vi "HW_7p1_Task2_nguyejk.vi"() -> ()   [LabVIEW 2016]
panel:
  out "Hypotension":dbl
  out "Normal":dbl
  out "Hypertension":dbl
  in  "Numeric":i32
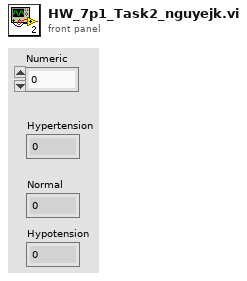
[diagram p1: front panel]
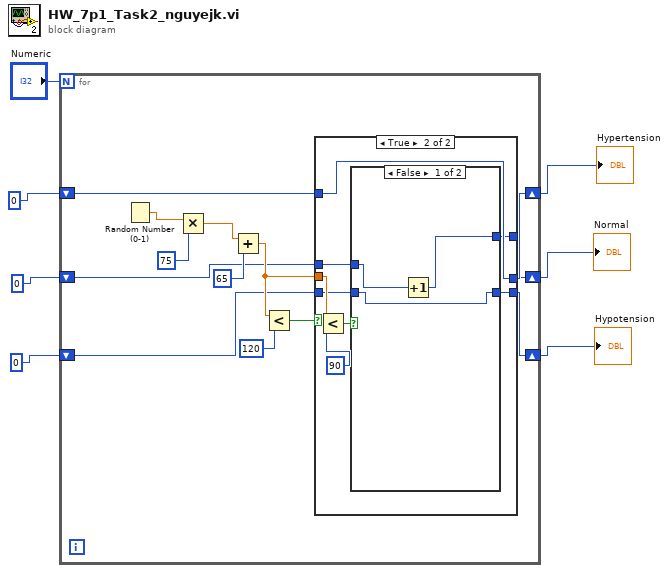
[diagram p0: block diagram]
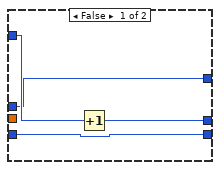
[diagram p2: hidden frame]
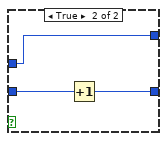
[diagram p3: hidden frame]
diagram:
  n1 = for {
    N: "Numeric" -> [_]
    shift-right: [w14] -> w4
    shift-left: 0 -> [w12]
    shift-right: [w11] -> w5
    shift-left: 0 -> [w10]
    shift-right: [w9] -> w1
    shift-left: 0 -> [w8]
    n2 = Random Number (0-1)() -> (number: 0 to 1=w17:dbl)
    n3 = Multiply(x=w17, y=75) -> (x*y=w19:dbl)
    n4 = Add(x=w19, y=65) -> (x+y=w13:dbl)
    n5 = Less?(x=w13, y=120) -> (x < y?=w16:bool)
    n6 = case shown="True" w16 {
      tunnel: [w24 w29] -> w14
      tunnel: w13 -> [_ w31]
      tunnel: w12 -> [w23 w29]
      tunnel: [w21 w28] -> w11
      tunnel: w10 -> [w21 w27]
      tunnel: [w22 w26] -> w9
      tunnel: w8 -> [w22 w25]
      frame False {
        n7 = Increment(x=w23) -> (x+1=w24:i32)
      }
      frame True {
        n8 = Less?(x=w31, y=90) -> (x < y?=w30:bool)
        n9 = case shown="False" w30 {
          tunnel: [w33 w38] -> w28
          tunnel: w27 -> [w33 w37]
          tunnel: [w35 w36] -> w26
          tunnel: w25 -> [w34 w36]
          frame False {
            n10 = Increment(x=w34) -> (x+1=w35:i32)
          }
          frame True {
            n11 = Increment(x=w37) -> (x+1=w38:i32)
          }
        }
      }
    }
  }
  "Hypertension" <- w4
  "Normal" <- w1
  "Hypotension" <- w5
